vi "ETH2_SOF Check.vi"(11 "Bytes data in":u8[](array[numeric])) -> (3 "index of passed smpl":i32[](array[numeric]))   [LabVIEW 2022 SP3]
panel:
  out "Passed samples":i32
  out "Numeric":i32
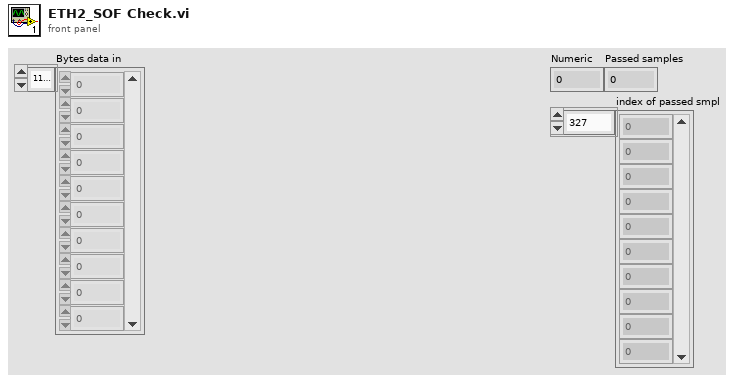
[diagram p1: front panel]
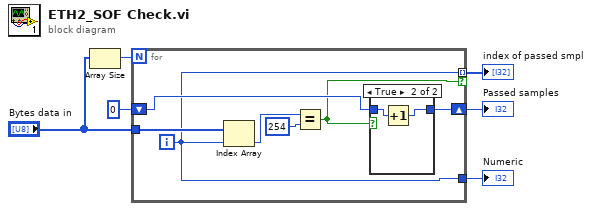
[diagram p0: block diagram]
diagram:
  n1 = Array Size(array="Bytes data in") -> (size(s)=w1:i32)
  n2 = for {
    N: w1 -> [_]
    tunnel: "Bytes data in" -> [w13]
    shift-right: [w9] -> w3
    shift-left: 0 ("x") -> [w10]
    tunnel: [w7] -> w4 mode=indexing if=w8
    tunnel: [w7] -> w5
    i -> [w7]
    n3 = Index Array(array=w13, index=w7) -> (element=w12:u8)
    n4 = Equal?(x=w12, y=u8 254) -> (x = y?=w8:bool)
    n5 = case shown="True" w8 {
      tunnel: w10 -> [w14 w16]
      tunnel: [w14 w15] -> w9
      frame False {
      }
      frame True {
        n6 = Increment(x=w16) -> (x+1=w15:i32)
      }
    }
  }
  "Numeric" <- w5
  "index of passed smpl" <- w4
  "Passed samples" <- w3
